vi "PV_Core_Fmt_GetSaphirApplicationPseudo.vi"(8 "error in":errorcluster) -> (0 "error out":errorcluster, 3 "Pseudo":string="XXX")   [LabVIEW 2020]
panel:
  # "Input"
  # "Output"
  # "Local"
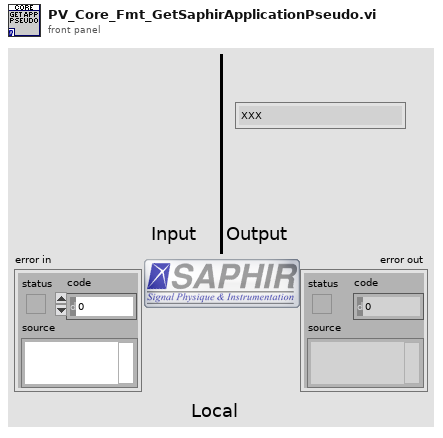
[diagram p1: front panel]
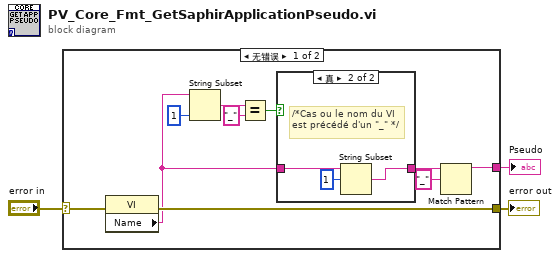
[diagram p0: block diagram]
diagram:
  n1 = case shown="无错误" "error in" {
    selector: "error in" -> [w12 w18]
    tunnel: [w11 w18] -> w2
    tunnel: [w10 _] -> w1
    frame No Error {
      n2 = property class="VI"(error in=w12) -> (error out=w11:errorcluster, "Name"=w6:string)  [unwired: 1 in, 1 out]
      n3 = String Subset(string=w6, length (rest)=1 ("length (rest)")) -> (substring=w8:string)  [unwired: 1 out]
      n4 = Equal?(x=w8, y="_" ("regular expression")) -> (x = y?=w4:bool)
      n5 = case shown="真" w4 {
        tunnel: w6 -> [w14 w16]
        tunnel: [w14 w15] -> w5
        frame False {
        }
        frame True {
          # "/*Cas ou le nom du VI est précédé d'un \"_\" */"
          n6 = String Subset(string=w16, offset (0)=1 ("length (rest)")) -> (substring=w15:string)  [unwired: 1 out]
        }
      }
      n7 = Match Pattern(string=w5, regular expression="_") -> (before substring=w10:string)  [unwired: 4 out]
    }
    frame Error {
    }
  }
  "error out" <- w2
  "Pseudo" <- w1
